vi "G#Template_CreateBase.vi"(0 "reference in":refnum<class "G#Template.lvclass">, 5 "error in (no error)":errorcluster) -> (14 "reference out":refnum<class "G#Template.lvclass">, 19 "error out":errorcluster)   [LabVIEW 2020, in "G#Template.lvclass"]
doc: "Constructor."
uses:
  <vilib>/addons/_AddQ/G#Templates/G#Template/G#Template.lvclass
  C:/Program Files (x86)/National Instruments/LabVIEW 2020/vi.lib/addons/_AddQ/G#Object/G#Object.lvclass
  <vilib>/addons/_AddQ/G#Object/G#Object.lvclass
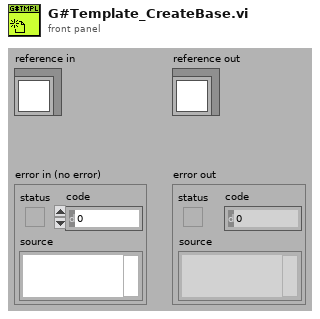
[diagram p1: front panel]
types:
  T1 = typedef "G#Template.lvclass/ObjectAttributesRef.ctl" = refnum<data-value>
  T2 = typedef "G#Template.lvclass/ObjectAttributes.ctl" = cluster{"MyAttribute":dbl}
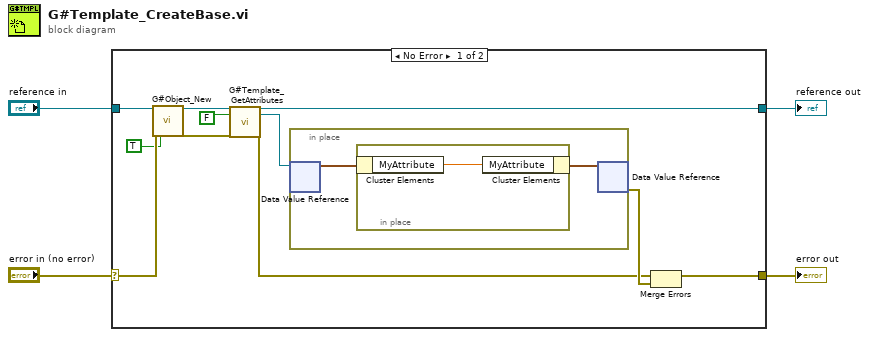
[diagram p0: block diagram]
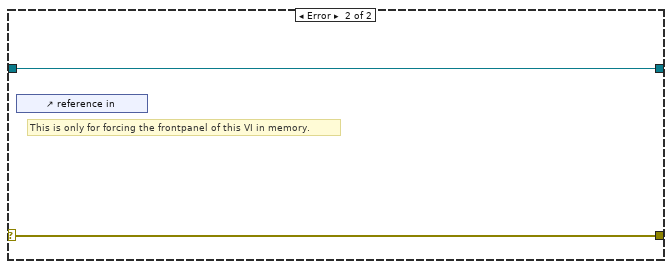
[diagram p2: hidden frame]
diagram:
  n1 = case shown="No Error" "error in (no error)" {
    selector: "error in (no error)" -> [w14 w20]
    tunnel: [w6 w20] -> w3
    tunnel: [w5 w19] -> w1
    tunnel: "reference in" -> [w15 w19]
    frame No Error {
      n2 = call <vilib>:"G#Object_New.vi"("reference in"=w15, "error in (no error)"=w14, "user counter (T)?"=TRUE ("User Counter")) -> ("reference out"=w11:refnum<class "G#Template.lvclass">, "error out"=w10:errorcluster)  [unwired: 14 in, 1 out]
      n3 = call <vilib>:"G#Template_GetAttributes.vi"("reference in"=w11, "return data? (T)"=FALSE ("return data"), "error in (no error)"=w10) -> ("reference out"=w5:refnum<class "G#Template.lvclass">, "attributes ref"=w9:T1, "error out"=w7:errorcluster)  [unwired: 13 in, 1 out]
      n4 = in-place {
        n5 = in-place-dvr #1(w9) -> (w16:T2)  [unwired: 1 out]
        n6 = in-place {
          n7 = in-place-cluster #2(w16) -> ("MyAttribute"=w18:dbl)
          n8 = in-place-cluster #2("MyAttribute"=w18) -> (w17:T2)
        }
        n9 = in-place-dvr #1(w17) -> (w12:errorcluster)  [unwired: 1 out]
      }
      n10 = Merge Errors(w7, w12) -> (w6:errorcluster)
    }
    frame Error {
      # "This is only for forcing the frontpanel of this VI in memory."
      n11 = control-ref of="reference in"() -> ()  [unwired: 1 out]
    }
  }
  "error out" <- w3
  "reference out" <- w1
